vi "CreateVIMInstanceConnections.vi"(8 "error in (no error)":errorcluster, 11 "CDependencyList in":refnum<class "CDependencyList.lvclass">) -> (0 "error out":errorcluster, 3 "CDependencyList out":refnum<class "CDependencyList.lvclass">)   [LabVIEW 2020, in "DependencyInspection.lvlib" / "CDependencyList.lvclass"]
uses:
  CDependencyList/CDependencyList.lvclass
  LabVIEWObjectInterfaces/ILabVIEWItem/ILabVIEWItem.lvclass
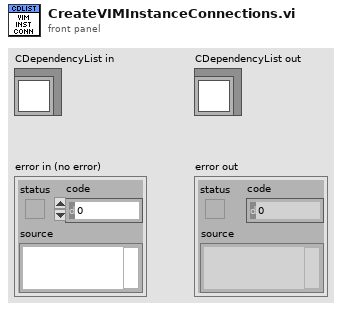
[diagram p1: front panel]
types:
  T1 = typedef "DependencyInspection.lvlib/CDependencyList.lvclass/DependencyListRef.ctl" = refnum<data-value>
  T2 = typedef "DependencyInspection.lvlib/CDependencyList.lvclass/DependencyList.ctl" = map{string, refnum<class "ILabVIEWItem.lvclass">}
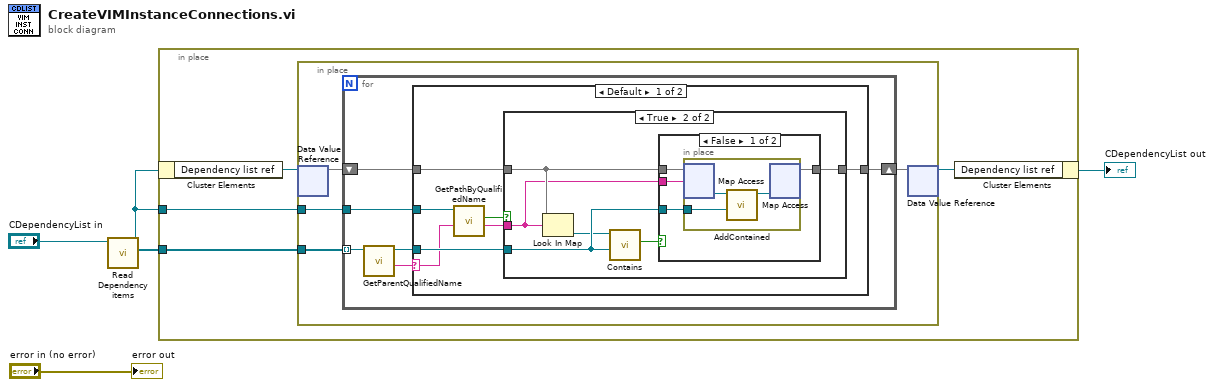
[diagram p0: block diagram]
diagram:
  n1 = call-dynamic "Read Dependency items.vi"("CDependencyList in"="CDependencyList in") -> ("Dependency items"=w1:refnum<class "ILabVIEWItem.lvclass">[], "CDependencyList out"=w2:refnum<class "CDependencyList.lvclass">)  [unwired: 9 in]
  n2 = in-place {
    in-place-border: w2 -> [w7]
    in-place-border: w1 -> [w6]
    n3 = in-place-cluster #1(w2) -> ("Dependency list ref"=w9:T1)
    n4 = in-place {
      in-place-border: w7 -> [w11]
      in-place-border: w6 -> [w10]
      n5 = in-place-dvr #2(w9) -> (w12:T2)  [unwired: 1 out]
      n6 = for {
        shift-right: [w16] -> w13
        shift-left: w12 -> [w17]
        tunnel: w11 -> [w15]
        tunnel: w10 -> [w14] mode=indexing
        n7 = call-dynamic "GetParentQualifiedName.vi"("ILabVIEWItem in"=w14) -> ("Name"=w19:string, "ILabVIEWItem out"=w18:refnum<class "ILabVIEWItem.lvclass">)  [unwired: 8 in, 1 out]
        n8 = case shown="Default" w19 {
          selector: w19 -> [w22 _]
          tunnel: w18 -> [w25 _]
          tunnel: w17 -> [w26 w42]
          tunnel: [w24 w42] -> w16
          tunnel: w15 -> [w23 _]
          frame Default {
            n9 = call-dynamic "GetPathByQualifiedName.vi"("Qualified name"=w22, "CDependencyList in"=w23) -> ("Path"=w20:string, "key found?"=w21:bool)  [unwired: 6 in, 2 out]
            n10 = case shown="True" w21 {
              tunnel: w20 -> [_ w29]
              tunnel: w26 -> [w27 w30]
              tunnel: w25 -> [_ w31]
              tunnel: [w27 w32] -> w24
              frame False {
              }
              frame True {
                n11 = Look In Map(map=w30, key=w29) -> (value=w28:refnum<class "ILabVIEWItem.lvclass">)  [unwired: 1 in, 1 out]
                n12 = call-dynamic "Contains.vi"("Item"=w31, "ILabVIEWItem in"=w28) -> ("Contains?"=w33:bool)  [unwired: 7 in, 2 out]
                n13 = case shown="False" w33 {
                  tunnel: w30 -> [w35 w41]
                  tunnel: [w34 w41] -> w32
                  tunnel: w29 -> [w37 _]
                  tunnel: w31 -> [w36 _]
                  frame False {
                    n14 = in-place {
                      in-place-border: w36 -> [w39]
                      n15 = in-place-map #3(w35, w37) -> (w40:refnum<class "ILabVIEWItem.lvclass">)  [unwired: 1 in, 1 out]
                      n16 = call-dynamic "AddContained.vi"("Item to contain"=w39, "ILabVIEWItem in"=w40) -> ("ILabVIEWItem out"=w38:refnum<class "ILabVIEWItem.lvclass">)  [unwired: 7 in, 2 out]
                      n17 = in-place-map #3(w38) -> (w34:T2)  [unwired: 1 in, 2 out]
                    }
                  }
                  frame True {
                  }
                }
              }
            }
          }
          frame "" {
          }
        }
      }
      n18 = in-place-dvr #2(w13) -> (w8:T1)  [unwired: 1 out]
    }
    n19 = in-place-cluster #1("Dependency list ref"=w8) -> (→"CDependencyList out":refnum<class "CDependencyList.lvclass">)
  }
  "error out" <- "error in (no error)"
